vi "InitVolumeAndPressureRatioSamples.vi"   [LabVIEW 2013]
uses:
  GlobalVariables/VolumeAndPressureRatioSamples.vi
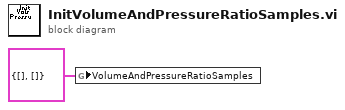
[diagram p0: block diagram]
diagram:
  n1 = global write "VolumeAndPressureRatioSamples.vi" "VolumeAndPressureRatioSamples"(cluster{"PressureRatios":dbl[], "Volumes":dbl[]} {"PressureRatios"=[], "Volumes"=[]} ("VolumeAndPressureRatioSamples")) -> ()
